vi "IMAQ Example.vi"() -> ()   [LabVIEW 2020]
uses:
  g_industrial_cam/Camera/Camera.lvclass
  g_industrial_cam/Buffer/Buffer.lvclass
panel:
  in  "Bit Depth":enum16{"Mono10", "Mono8"}(ring)
  out "Copy Array":T1(plugin-control)
  out "Byte Stream":T1(plugin-control)
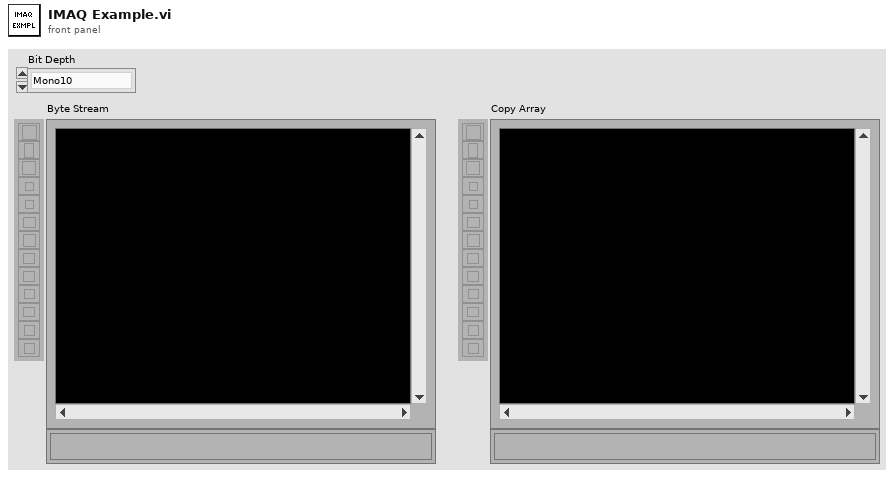
[diagram p1: front panel]
types:
  T1 = typedef "IMAQ Image.ctl" = refnum<image>
  T2 = typedef "Device Enumeration.ctl" = cluster{"ID":string, "Protocol":string, "Vendor":string, "Model":string, "Serial":string, "Address":string}
  T3 = typedef "Image Type" = u32
  T4 = typedef "Buffer.lvclass/Image Size.ctl" = cluster{"Width":u16, "Height":u16}
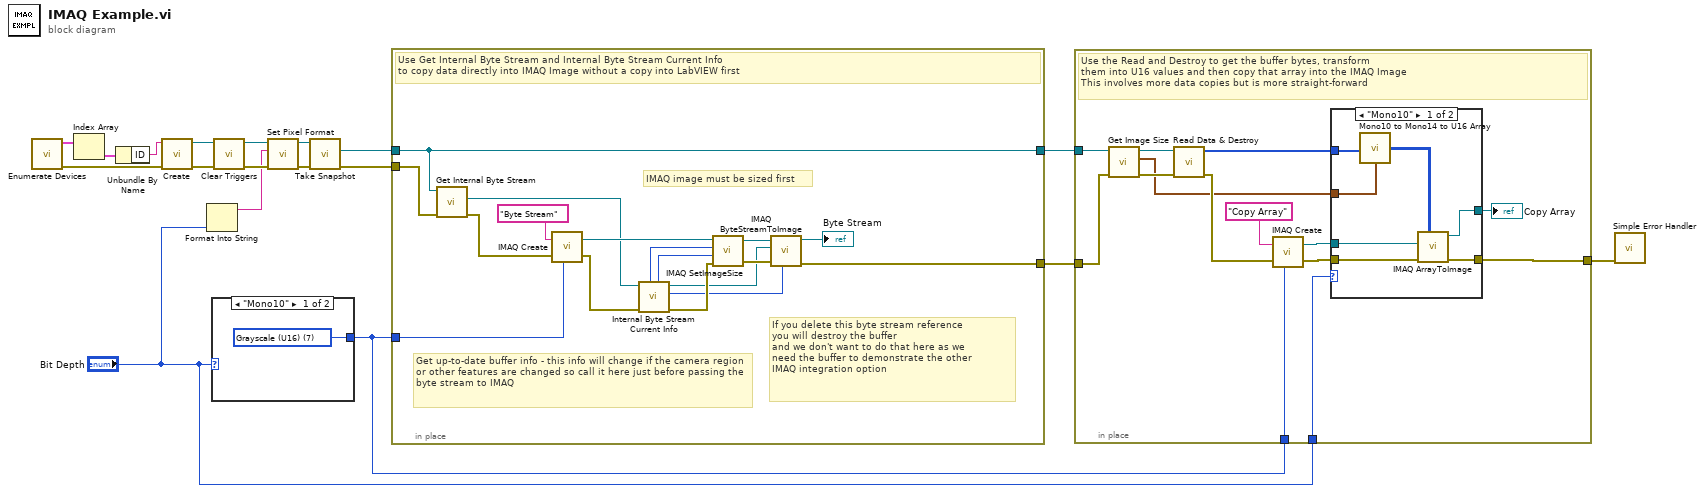
[diagram p0: block diagram]
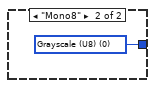
[diagram p2: hidden frame]
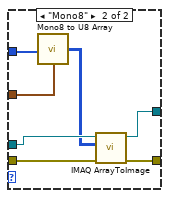
[diagram p3: hidden frame]
diagram:
  n1 = call "Enumerate Devices.vi"() -> ("error out"=w16:errorcluster, "Devices"=w18:T2[])  [unwired: 10 in]
  n2 = Index Array(array=w18) -> (element=w17:T2)  [unwired: 1 in]
  n3 = Unbundle By Name(w17) -> ("ID"=w15:string)
  n4 = call "Create.vi"("error in (no error)"=w16, "Identifier (ID, IP etc)"=w15) -> ("error out"=w14:errorcluster, "Camera"=w13:refnum<class "Camera.lvclass">)  [unwired: 8 in]
  n5 = Format Into String("Bit Depth") -> (resulting string=w3:string)  [unwired: 3 in, 1 out]
  n6 = case shown="\"Mono10\"" "Bit Depth" {
    tunnel: [w19 w20] -> w2
    frame "Mono10" {
      w19 = T3 7 items=["Grayscale (U8)", "Grayscale (I16)", "Grayscale (SGL)", "Complex (CSG)", "RGB (U32)", "HSL (U32)", "RGB (U64)", "Grayscale (U16)"] ("Image Type")
    }
    frame "Mono8" {
      w20 = T3 0 items=["Grayscale (U8)", "Grayscale (I16)", "Grayscale (SGL)", "Complex (CSG)", "RGB (U32)", "HSL (U32)", "RGB (U64)", "Grayscale (U16)"] ("Image Type")
    }
  }
  n7 = call "Clear Triggers.vi"("error in (no error)"=w14, "Camera in"=w13) -> ("error out"=w12:errorcluster, "Camera"=w11:refnum<class "Camera.lvclass">)  [unwired: 8 in]
  n8 = call "Set Pixel Format.vi"("error in (no error)"=w12, "Pixel Format"=w3, "Camera in"=w11) -> ("error out"=w10:errorcluster, "Camera"=w9:refnum<class "Camera.lvclass">)  [unwired: 7 in]
  n9 = call "Take Snapshot.vi"("error in (no error)"=w10, "Camera in"=w9) -> ("error out"=w7:errorcluster, "New Buffer"=w8:refnum<class "Buffer.lvclass">)  [unwired: 7 in, 1 out]
  n10 = in-place {
    in-place-border: [w31] -> w5
    in-place-border: w8 -> [w22]
    in-place-border: w7 -> [w29]
    in-place-border: [w22] -> w6
    in-place-border: w2 -> [w21]
    # "If you delete this byte stream reference\nyou will destroy the buffer\nand we don't want to do that here as we\nneed the buffer to demonstrate the other\nIMAQ integration option"
    # "Get up-to-date buffer info - this info will change if the camera region or other features are changed so call it here just before passing the byte stream to IMAQ"
    # "IMAQ image must be sized first"
    # "Use Get Internal Byte Stream and Internal Byte Stream Current Info\nto copy data directly into IMAQ Image without a copy into LabVIEW first"
    n11 = call "Get Internal Byte Stream.vi"("error in (no error)"=w29, "Buffer Data in"=w22) -> ("error out"=w28:errorcluster, "Byte Stream"=w32:refnum<data-value>)  [unwired: 7 in, 1 out]
    n12 = call "IMAQ Create"("Image Name"="Byte Stream", "Image Type"=w21, "error in (no error)"=w28) -> ("New Image"=w34:T1, "error out"=w27:errorcluster)  [unwired: 2 in]
    n13 = call "Internal Byte Stream Current Info.vi"("error in (no error)"=w27, "Byte Stream in"=w32) -> ("error out"=w37:errorcluster, "Byte Stream Size (bytes)"=w26:u64, "Byte Stream"=w30:refnum<data-value>, "Y Resolution"=w24:i32, "X Resolution"=w25:i32)  [unwired: 3 in]
    n14 = call "IMAQ SetImageSize"("error in (no error)"=w37, "Y Resolution"=w24, "X Resolution"=w25, "Image"=w34) -> ("error out"=w36:errorcluster, "Image Out"=w33:T1)  [unwired: 1 in]
    n15 = call "IMAQ ByteStreamToImage"("Bytes to Copy"=w26, "error in (no error)"=w36, "Byte Stream In"=w30, "Image In"=w33) -> ("error out"=w31:errorcluster, "Image Out"=→"Byte Stream":T1)  [unwired: 3 in, 3 out]
  }
  n16 = in-place {
    in-place-border: w6 -> [w43]
    in-place-border: w5 -> [w46]
    in-place-border: [w40] -> w4
    in-place-border: w2 -> [w39]
    in-place-border: "Bit Depth" -> [w38]
    # "Use the Read and Destroy to get the buffer bytes, transform\nthem into U16 values and then copy that array into the IMAQ Image\nThis involves more data copies but is more straight-forward"
    n17 = call "Get Image Size.vi"("error in (no error)"=w46, "Buffer in"=w43) -> ("error out"=w44:errorcluster, "Image Size"=w41:T4, "Buffer"=w42:refnum<class "Buffer.lvclass">)  [unwired: 7 in]
    n18 = call "Read Data & Destroy.vi"("error in (no error)"=w44, "Buffer in"=w42) -> ("error out"=w45:errorcluster, "Data"=w51:u8[])  [unwired: 8 in]
    n19 = call "IMAQ Create"("Image Name"="Copy Array", "Image Type"=w39, "error in (no error)"=w45) -> ("New Image"=w49:T1, "error out"=w48:errorcluster)  [unwired: 2 in]
    n20 = case shown="\"Mono10\"" w38 {
      tunnel: w51 -> [w58 w65]
      tunnel: w49 -> [w57 w64]
      tunnel: w48 -> [w56 w63]
      tunnel: [w54 w62] -> w47
      tunnel: w41 -> [w53 w61]
      tunnel: [w52 w60] -> w40
      frame "Mono10" {
        n21 = call "Mono10 to Mono14 to U16 Array.vi"("2-Byte Mono Data"=w58, "Image Size"=w53) -> ("U16 Pixels"=w55:u16[][])
        n22 = call "IMAQ ArrayToImage"("Image Pixels (U16)"=w55, "error in (no error)"=w56, "Image"=w57) -> ("error out"=w52:errorcluster, "Image Out"=w54:T1)  [unwired: 7 in]
      }
      frame "Mono8" {
        n23 = call "Mono8 to U8 Array.vi"("1-Byte Mono Data"=w65, "Image Size"=w61) -> ("U8 Pixels"=w59:u8[][])
        n24 = call "IMAQ ArrayToImage"("error in (no error)"=w63, "Image Pixels (U8)"=w59, "Image"=w64) -> ("error out"=w60:errorcluster, "Image Out"=w62:T1)  [unwired: 7 in]
      }
    }
    "Copy Array" <- w47
  }
  n25 = call <vilib>:"Simple Error Handler.vi"("error in (no error)"=w4) -> ()  [unwired: 4 in, 5 out]
